vi "Model - Get Stop.vi"(8 "error in (no error)":errorcluster, 11 "View Model":T1) -> (0 "error out":errorcluster, 2 "Stop?":bool, 3 "View Model":T1)   [LabVIEW 2017]
doc: "Get actual Stop value from DVR"
uses:
  Controls/View Model.ctl
  Controls/Shared Model.ctl
  Error/Controls/Error Model.ctl
  Error/Controls/Error Event.ctl
  Error/Controls/Error Type.ctl
  Configuration/Controls/Config DB Model.ctl
  Configuration/Controls/Config DB Command.ctl
  Configuration/Controls/Config DB Record.ctl
  Controller/Controls/Controller Model.ctl
  Controller/Controls/Elevator Location.ctl
  Controller/Controls/Elevator Direction Event.ctl
  Controller/Controls/Elevator Direction.ctl
  Controller/Controls/Elevator CMD Event.ctl
  Controller/Controls/Elevator Commands.ctl
  Controller/Controls/Elevator Overhead.ctl
  Controller/Controls/Elevator State.ctl
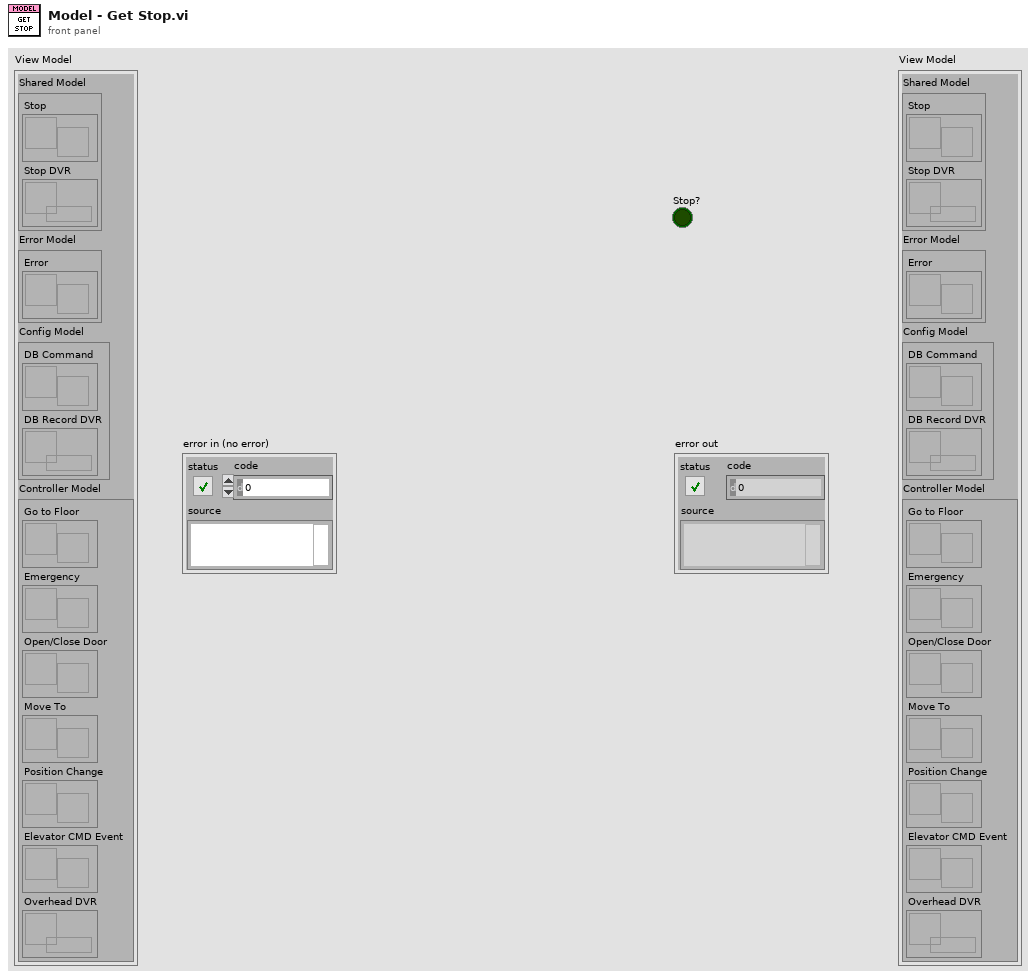
[diagram p1: front panel]
types:
  T1 = typedef "View Model.ctl" = cluster{"Shared Model":T2, "Error Model":T3, "Config Model":T4, "Controller Model":T5}
  T2 = typedef "Shared Model.ctl" = cluster{"Stop":refnum<user-event>, "Stop DVR":refnum<data-value>}
  T3 = typedef "Error Model.ctl" = cluster{"Error":refnum<user-event>}
  T4 = typedef "Config DB Model.ctl" = cluster{"DB Command":refnum<user-event>, "DB Record DVR":refnum<data-value>}
  T5 = typedef "Controller Model.ctl" = cluster{"Go to Floor":refnum<user-event>, "Emergency":refnum<user-event>, "Open/Close Door":refnum<user-event>, "Move To":refnum<user-event>, "Position Change":refnum<user-event>, "Elevator CMD Event":refnum<user-event>, "Overhead DVR":refnum<data-value>}
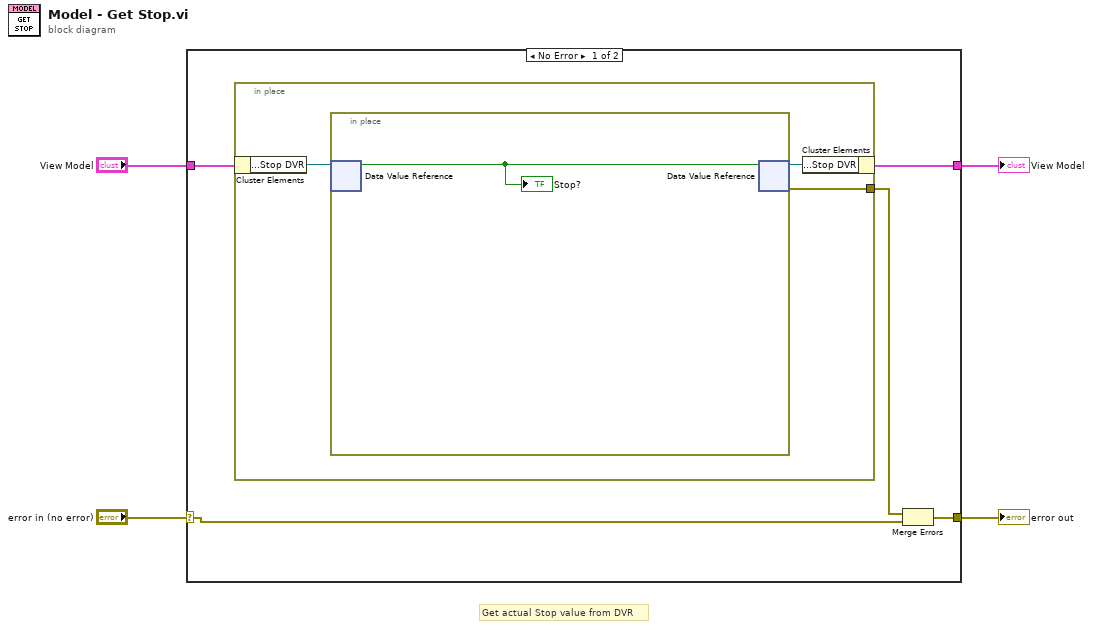
[diagram p0: block diagram]
diagram:
  # "Get actual Stop value from DVR"
  n1 = case shown="No Error" "error in (no error)" {
    selector: "error in (no error)" -> [w7 w14]
    tunnel: "View Model" -> [w9 w15]
    tunnel: [w8 w15] -> w2
    tunnel: [w6 w14] -> w1
    frame No Error {
      n2 = in-place {
        in-place-border: [w10] -> w5
        n3 = in-place-cluster #1(w9) -> ("Shared Model.Stop DVR"=w12:refnum<data-value>)
        n4 = in-place {
          n5 = in-place-dvr #2(w12) -> (w13:bool)  [unwired: 1 out]
          "Stop?" <- w13
          n6 = in-place-dvr #2(w13) -> (w11:refnum<data-value>, w10:errorcluster)
        }
        n7 = in-place-cluster #1("Shared Model.Stop DVR"=w11) -> (w8:T1)
      }
      n8 = Merge Errors(w5, w7) -> (w6:errorcluster)
    }
    frame Error {
    }
  }
  "error out" <- w1
  "View Model" <- w2
